vi "Eleminate Deadband.vi"(1 "Axis In":dbl, 2 "Deadband":dbl) -> (0 "Axis Out":dbl)   [LabVIEW 2016]
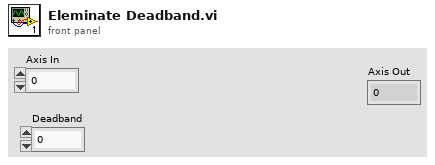
[diagram p1: front panel]
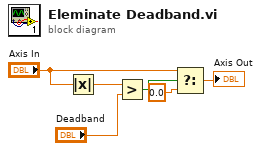
[diagram p0: block diagram]
diagram:
  n1 = Absolute Value(x="Axis In") -> (abs(x)=w5:dbl)
  n2 = Greater?(x=w5, y="Deadband") -> (0:w6:bool)
  n3 = Select(t="Axis In", s=w6, f=0.0) -> (s? t:f=→"Axis Out":dbl)
